vi "输入数据判定.vi"(7 "主从选择":u16(ring) items=["主板", "从板"], 8 "主板选项":string="项目信息", 9 "进度引用":refnum<vi>, 10 "从板个数":dbl=1.0, 11 "错误代码":u32) -> ()   [LabVIEW 2013]
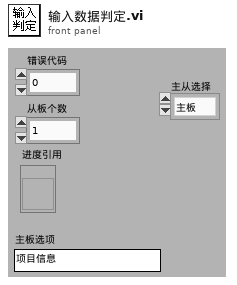
[diagram p1: front panel]
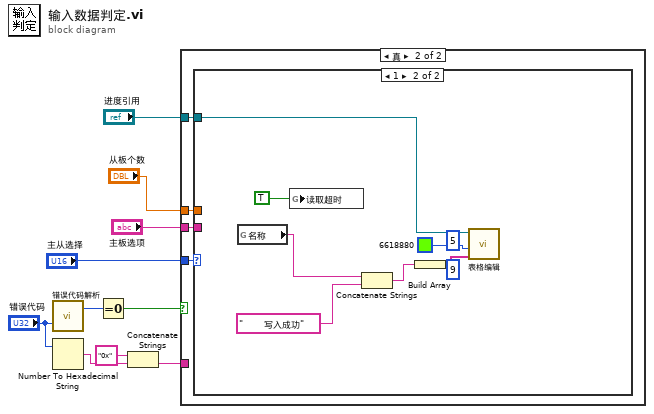
[diagram p0: block diagram]
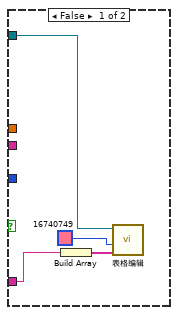
[diagram p2: hidden frame]
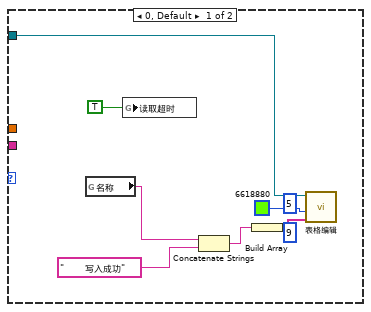
[diagram p3: hidden frame]
diagram:
  n1 = call "错误代码解析.vi"("错误代码"="错误代码") -> ("错误代码"=w6:i32)  [unwired: 2 out]
  n2 = Number To Hexadecimal String(2:"错误代码") -> (0:w4:string)  [unwired: 1 out]
  n3 = Equal To 0?(x=w6) -> (x = 0?=w7:bool)
  n4 = Concatenate Strings("0x" ("字符串"), w4) -> (w3:string)
  n5 = case shown="真" w7 {
    tunnel: "主板选项" -> [_ w18]
    tunnel: "进度引用" -> [w11 w17]
    tunnel: "从板个数" -> [_ w16]
    tunnel: "主从选择" -> [_ w15]
    tunnel: w3 -> [w14 _]
    frame False {
      n6 = Build Array(w14) -> (w13:string[])
      n7 = call "表格编辑.vi"("新元素/子数组"=w13, "活动单元格:单元格背景色"=u32 16740749, "MCListbox引用句柄"=w11) -> ()  [unwired: 9 out]
    }
    frame True {
      n8 = case shown="1" w15 {
        tunnel: w18 -> [_ _]
        tunnel: w17 -> [w21 w28]
        tunnel: w16 -> [_ _]
        frame 0, Default {
          (unwired) u32 9 ("表格总行数")
          (unwired) 5 ("保留行数")
          n9 = global read "全局 1.vi" "名称"() -> (w19:string)
          n10 = global write "EV05全局变量1.vi" "读取超时"(TRUE ("读取超时")) -> ()
          n11 = Concatenate Strings(w19, "       写入成功" ("字符串")) -> (w24:string)
          n12 = Build Array(w24) -> (w23:string[])
          n13 = call "表格编辑.vi"("新元素/子数组"=w23, "活动单元格:单元格背景色"=u32 6618880, "MCListbox引用句柄"=w21) -> ()  [unwired: 9 out]
        }
        frame 1 {
          (unwired) u32 9 ("表格总行数")
          (unwired) 5 ("保留行数")
          n14 = global read "全局 1.vi" "名称"() -> (w26:string)
          n15 = global write "EV05全局变量1.vi" "读取超时"(TRUE ("读取超时")) -> ()
          n16 = Concatenate Strings(w26, "       写入成功" ("字符串")) -> (w31:string)
          n17 = Build Array(w31) -> (w30:string[])
          n18 = call "表格编辑.vi"("新元素/子数组"=w30, "活动单元格:单元格背景色"=u32 6618880, "MCListbox引用句柄"=w28) -> ()  [unwired: 9 out]
        }
      }
    }
  }
